vi "Insert Coin.vi"(0 "reference in":refnum<class "Has Coin State.lvclass">, 5 "error in (no error)":errorcluster) -> (14 "reference out":refnum<class "Has Coin State.lvclass">, 19 "error out":errorcluster)   [LabVIEW 2013, in "Has Coin State.lvclass"]
uses:
  Has Coin State.lvclass
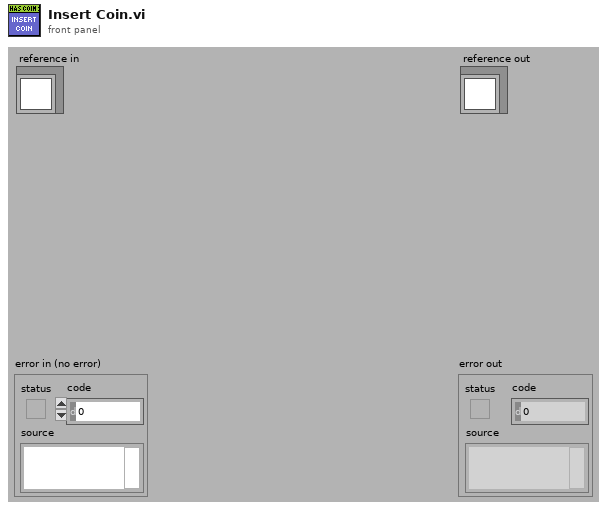
[diagram p1: front panel]
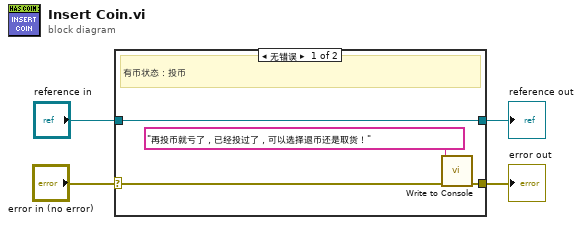
[diagram p0: block diagram]
diagram:
  n1 = case shown="无错误" "error in (no error)" {
    selector: "error in (no error)" -> [w7 w10]
    tunnel: [w5 w10] -> w3
    tunnel: [w8 w9] -> w1
    tunnel: "reference in" -> [w8 w9]
    frame No Error {
      # "有币状态：投币"
      n2 = call "Write to Console.vi"("error in (no error)"=w7, "Input"="再投币就亏了，已经投过了，可以选择退币还是取货！") -> ("error out"=w5:errorcluster)  [unwired: 9 in]
    }
    frame Error {
    }
  }
  "error out" <- w3
  "reference out" <- w1
